vi "Visor.vi"(1 "Line IN":T1) -> (0 "Line OUT":T1)   [LabVIEW 2015]
uses:
  <vilib>/NXT/Subs/LVHSConnector.ctl
  <vilib>/NXT/LegoClasses/BrickReference/BrickReference.lvclass
  <vilib>/NXT/Block Support/NXT_InputPort.ctl
  <vilib>/NXT/Dual Mode Library/Sensors/Sound_dBA.vi
  <vilib>/NXT/Dual Mode Library/Display/drawText_Center.vi
  <vilib>/NXT/Dual Mode Library/Sensors/Light_On.vi
  <vilib>/NXT/Dual Mode Library/Sensors/EV3_Ultrasonic_CM.vi
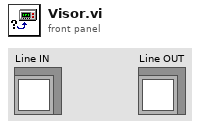
[diagram p1: front panel]
types:
  T1 = typedef "LVHSConnector.ctl" = refnum<class "BrickReference.lvclass">
  T2 = typedef "NXT_InputPort.ctl" = u32
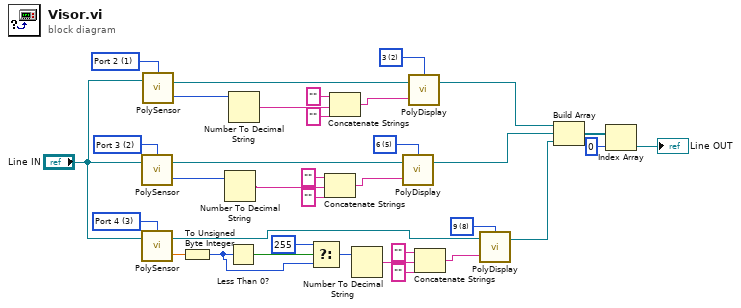
[diagram p0: block diagram]
diagram:
  w27 = T2 1 items=["Port 1", "Port 2", "Port 3", "Port 4"] ("Port (Port 2)")
  w26 = T2 2 items=["Port 1", "Port 2", "Port 3", "Port 4"] ("Port (Port 3)")
  w25 = T2 3 items=["Port 1", "Port 2", "Port 3", "Port 4"] ("Port (Port 1)")
  w22 = i16 8 items=["1", "2", "3", "4", "5", "6", "7", "8", "9", "10", "11", "12"] ("Line")
  w21 = i16 5 items=["1", "2", "3", "4", "5", "6", "7", "8", "9", "10", "11", "12"] ("Line")
  w20 = i16 2 items=["1", "2", "3", "4", "5", "6", "7", "8", "9", "10", "11", "12"] ("Line")
  n1 = call-poly <vilib>:"PolySensor.vi"("NXT/EV3"="Line IN", "Port (Port 3)"=w26) -> ("Scaled Value"=w10:i16, "NXT/EV3"=w23:T1)  [unwired: 1 in]
  n2 = call-poly <vilib>:"PolySensor.vi"("NXT/EV3"="Line IN", "Port (Port 1)"=w25) -> ("Centimeters"=w14:sgl, "NXT/EV3"=w24:T1)  [unwired: 1 in]
  n3 = call-poly <vilib>:"PolySensor.vi"("NXT/EV3"="Line IN", "Port (Port 2)"=w27) -> ("sound (dBA)"=w2:i16, "NXT/EV3"=w18:T1)  [unwired: 1 in]
  n4 = To Unsigned Byte Integer(number=w14) -> (unsigned 8bit integer=w17:u8)
  n5 = Number To Decimal String(number=w10) -> (decimal integer string=w11:string)  [unwired: 1 in]
  n6 = Less Than 0?(x=w17) -> (x < 0?=w15:bool)
  n7 = Number To Decimal String(number=w2) -> (decimal integer string=w12:string)  [unwired: 1 in]
  n8 = Select(t=u8 255, s=w15, f=w17) -> (s? t:f=w13:u8)
  n9 = Concatenate Strings("" ("string"), w11, "" ("string")) -> (w29:string)
  n10 = Concatenate Strings("" ("string"), w12, "" ("string")) -> (w19:string)
  n11 = Number To Decimal String(number=w13) -> (decimal integer string=w5:string)  [unwired: 1 in]
  n12 = call-poly <vilib>:"PolyDisplay.vi"("Text"=w29, "NXT/EV3"=w23, "Line"=w21) -> ("NXT/EV3"=w31:T1)  [unwired: 1 in]
  n13 = call-poly <vilib>:"PolyDisplay.vi"("Text"=w19, "NXT/EV3"=w18, "Line"=w20) -> ("NXT/EV3"=w30:T1)  [unwired: 1 in]
  n14 = Concatenate Strings("" ("string"), w5, "" ("string")) -> (w28:string)
  n15 = call-poly <vilib>:"PolyDisplay.vi"("Text"=w28, "NXT/EV3"=w24, "Line"=w22) -> ("NXT/EV3"=w32:T1)  [unwired: 1 in]
  n16 = Build Array(w30, w31, w32) -> (w33:T1[])
  n17 = Index Array(array=w33, index=0) -> (element=→"Line OUT":T1)
